vi "Update Mirror NP.vi"(8 "error in (no error)":errorcluster, 11 "Flip Mirror Containter in":refnum<class "Flip Mirror Containter.lvclass">) -> (0 "error out":errorcluster, 2 "Mirrors-NP":T1, 3 "Flip Mirror Containter out":refnum<class "Flip Mirror Containter.lvclass">)   [LabVIEW 2016]
uses:
  Classes/FlipMir/Flip Mirror Containter.lvclass
  Controls/Flip Mirrors.ctl
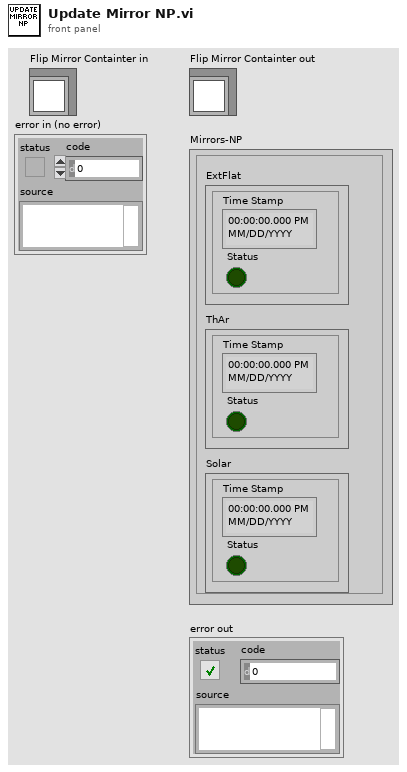
[diagram p1: front panel]
types:
  T1 = typedef "Flip Mirrors.ctl" = cluster{"Solar":cluster{"Status":bool, "Time Stamp":timestamp}, "ExtFlat":cluster{"Status":bool, "Time Stamp":timestamp}, "ThAr":cluster{"Status":bool, "Time Stamp":timestamp}}
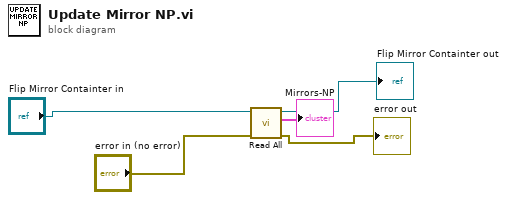
[diagram p0: block diagram]
diagram:
  n1 = call-dynamic "Read All.vi"("error in (no error)"="error in (no error)", "Flip Mirror Containter in"="Flip Mirror Containter in") -> ("error out"=→"error out":errorcluster, "Mirrors-NP"=→"Mirrors-NP":T1, "Flip Mirror Containter out"=→"Flip Mirror Containter out":refnum<class "Flip Mirror Containter.lvclass">)  [unwired: 7 in]
